vi "onHttpHead.vi"(6 "timeout":i32=10000, 8 "error in":errorcluster, 10 "url":string, 11 "http-client in":refnum<class "basic-http-client.lvclass">) -> (0 "error out":errorcluster, 2 "headers":string, 3 "http-client out":refnum<class "basic-http-client.lvclass">)   [LabVIEW 2025, in "basic-http-client.lvclass"]
uses:
  basic-http-client.lvclass
  basic-http-client.lvclass/basic-http-client.ctl
  <vilib>/httpClient/LabVIEWHTTPClient.lvlib
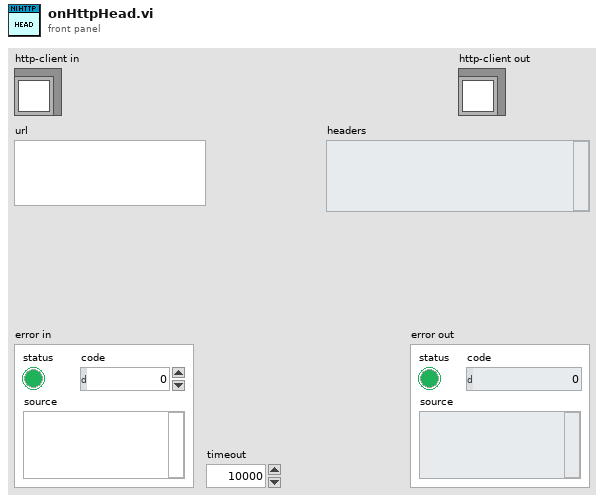
[diagram p1: front panel]
types:
  T1 = typedef "LabVIEWHTTPClient.lvlib/ClientHandle.ctl" = refnum<k1>
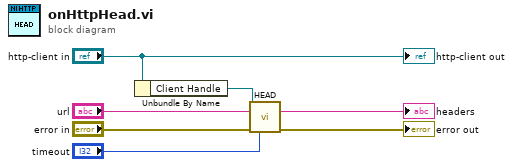
[diagram p0: block diagram]
diagram:
  n1 = Unbundle By Name("http-client in") -> ("Client Handle"=w2:T1)
  n2 = call <vilib>:"HEAD.vi"("client handle"=w2, "url"="url", "error in (no error)"="error in", "timeout (10000)"="timeout") -> ("headers"=→"headers":string, "error out"=→"error out":errorcluster)  [unwired: 9 in, 1 out]
  "http-client out" <- "http-client in"
